vi "ReferencedVariables_ReadReferencedVariable_4x4x4_Singleton.vi"(8 "error in (no error)":errorcluster) -> (0 "error out":errorcluster, 2 "ReplaceWithtypeDef":dbl)   [LabVIEW 2010]
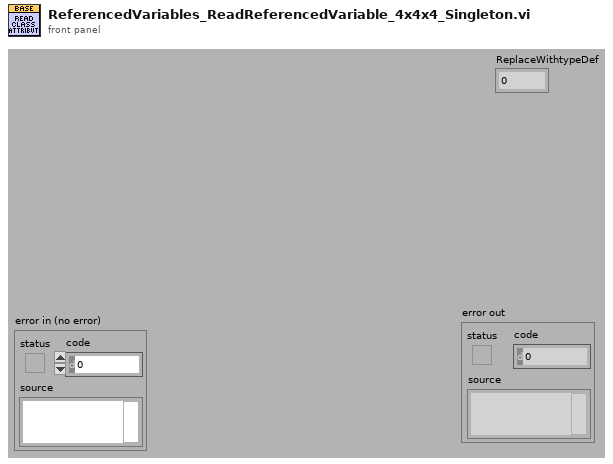
[diagram p1: front panel]
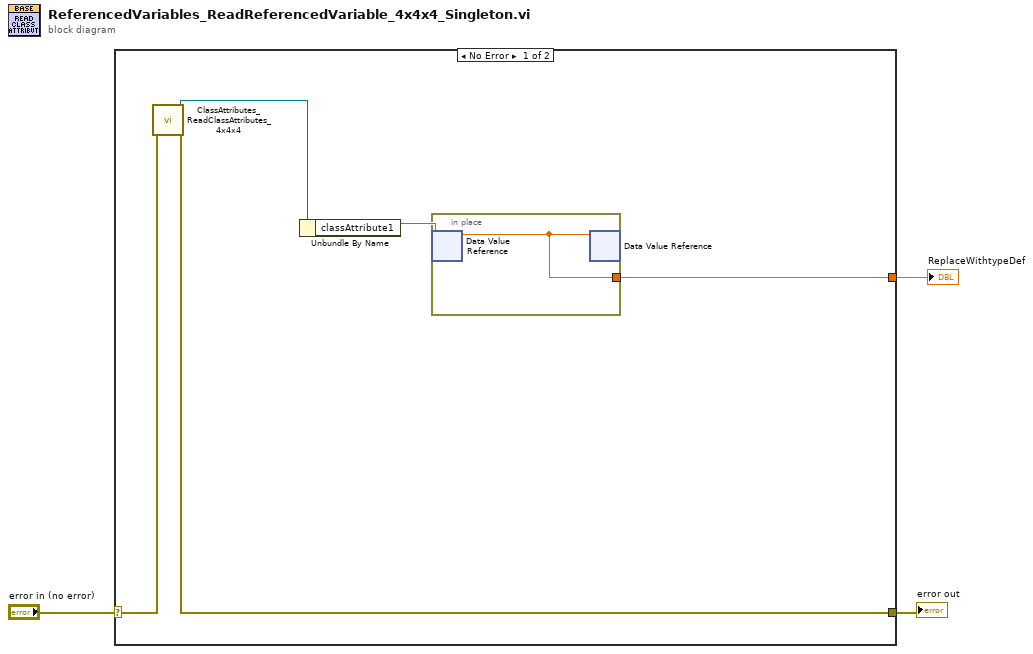
[diagram p0: block diagram]
diagram:
  n1 = case shown="No Error" "error in (no error)" {
    selector: "error in (no error)" -> [w8 w10]
    tunnel: [w5 w10] -> w2
    tunnel: [w4 _] -> w1
    frame No Error {
      n2 = call "ClassAttributes_ReadClassAttributes_4x4x4.vi"("error in (no error)"=w8) -> ("error out"=w5:errorcluster, "reference out"=w6:refnum<class>)  [unwired: 9 in]
      n3 = Unbundle By Name(w6) -> ("classAttribute1"=w7)
      n4 = in-place {
        in-place-border: [w9] -> w4
        n5 = in-place-dvr #1(w7) -> (w9:dbl)  [unwired: 1 out]
        n6 = in-place-dvr #1(w9) -> ()  [unwired: 2 out]
      }
    }
    frame Error {
    }
  }
  "error out" <- w2
  "ReplaceWithtypeDef" <- w1
